vi "Next.vi"(8 "error in (no error)":errorcluster, 11 "Vector in":refnum<class "Vector Parent.lvclass">) -> (0 "error out":errorcluster, 2 "Last?":bool, 3 "Vector out":refnum<class "Vector Parent.lvclass">)   [LabVIEW 2021, in "Vector Parent.lvclass"]
uses:
  Vector Parent.lvclass
  Vector Parent.lvclass/Vector Parent.ctl
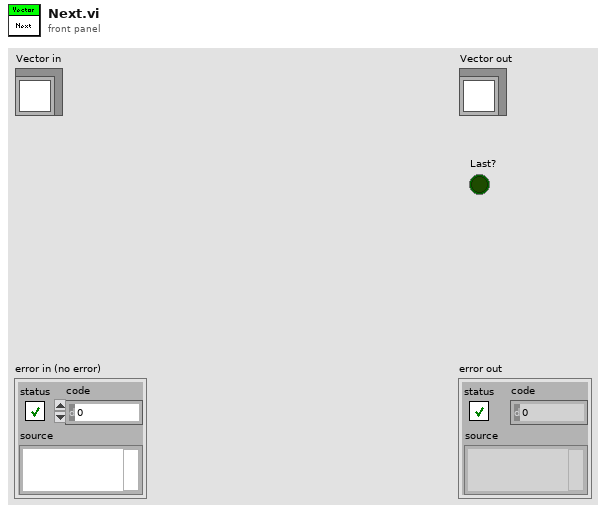
[diagram p1: front panel]
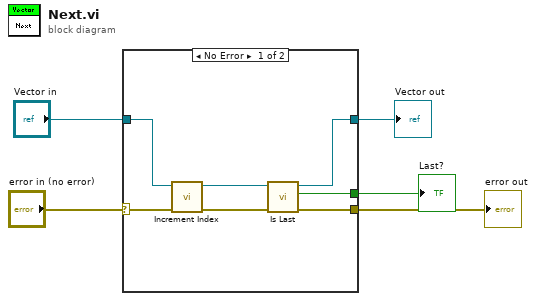
[diagram p0: block diagram]
diagram:
  n1 = case shown="No Error" "error in (no error)" {
    selector: "error in (no error)" -> [w6 w13]
    tunnel: [w12 w14] -> w5
    tunnel: [w11 _] -> w4
    tunnel: [w10 w13] -> w3
    tunnel: "Vector in" -> [w8 w14]
    frame No Error {
      n2 = call-dynamic "Increment Index.vi"("error in (no error)"=w6, "Vector Parent in"=w8) -> ("error out"=w7:errorcluster, "Vector Parent out"=w9:refnum<class "Vector Parent.lvclass">)  [unwired: 8 in]
      n3 = call-dynamic "Is Last.vi"("error in (no error)"=w7, "Vector in"=w9) -> ("error out"=w10:errorcluster, "Last?"=w11:bool, "Vector out"=w12:refnum<class "Vector Parent.lvclass">)  [unwired: 7 in]
    }
    frame Error {
    }
  }
  "error out" <- w3
  "Vector out" <- w5
  "Last?" <- w4
